vi "Connection Manager (general TDT).vi"(2 "Parent VI":refnum<vi>, 7 "AO Endpoints":string[](array[string])=["Right", "Left"], 9 "AI Endpoints":string[](array[string])=["Probe Mic Left", "Cal Mic"], 11 "error in (no error)":errorcluster) -> (4 "TDT-Device Config":T3, 6 "Properties":T2, 8 "Canceled?":bool, 15 "error out":errorcluster)   [LabVIEW 2020]
uses:
  Utility VIs/Buttons/KCheckmarkBoolean 2.ctl
  Utility VIs/Controls/KTable/KTable.xctl
  PXI DAQ VIs/TDT VIs/Typedefs/TDT-Device Config.ctl
  PXI DAQ VIs/TDT VIs/Typedefs/TDT-Output source.ctl
  PXI DAQ VIs/TDT VIs/Typedefs/TDT-Device ID.ctl
  PXI DAQ VIs/TDT VIs/Typedefs/TDT-Input source.ctl
  EPhys/LV Source/Typedefs/EPhys-Hardware Properties.ctl
panel:
  out "button":bool
  in  "Test Button":bool
  in  "Use kill switch":T1
  in  "Input Table":u16(xcontrol)
  in  "Path":path
  in  "Output Table":u16(xcontrol)
  in  "Biosemi":T1
  in  "Input":enum16{"Front panel", "RA4LI", "RA16LI"}(ring)
  out "Image":enum32{"None", "RX6", "RZ5", "RZ6"}(tab)
  in  "Input source":u16(ring) items=["Front panel", "RA4LI", "RA16LI"]
  in  "Run on":u16(ring) items=["RZ5"]
  in  "Cancel":bool
  in  "OK":bool
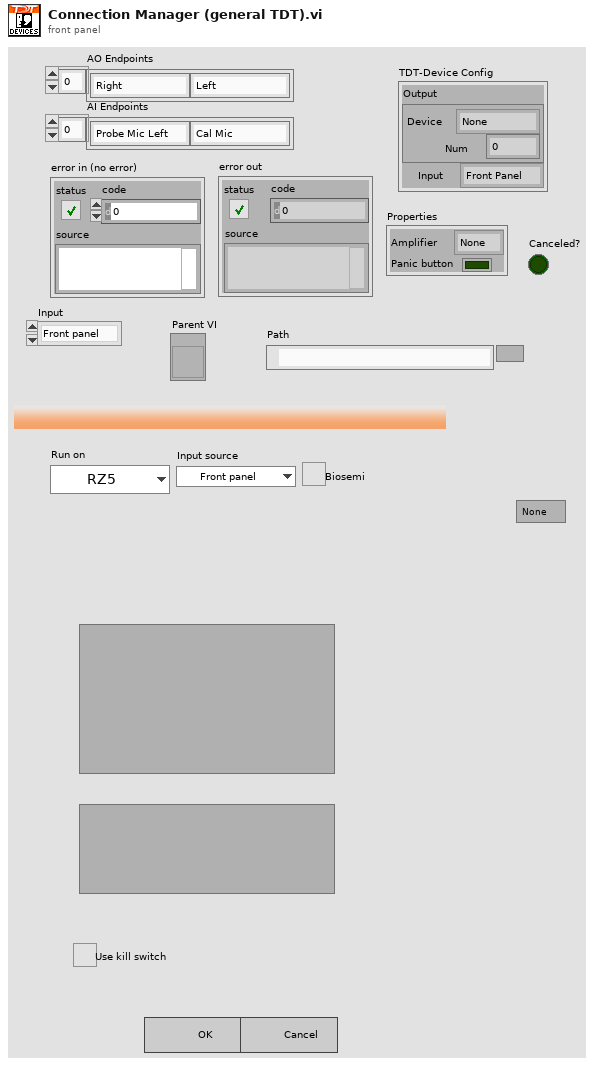
[diagram p1: front panel]
types:
  T1 = typedef "KCheckmarkBoolean 2.ctl" = bool
  T2 = typedef "EPhys-Hardware Properties.ctl" = cluster{"Amplifier":enum16{"None", "Biosemi", "Eclipse", "Eclipse (N.C.)", "Grass"}, "Panic button":bool}
  T3 = typedef "TDT-Device Config.ctl" = cluster{"Output":T4, "Input":T6}
  T4 = typedef "TDT-Output source.ctl" = cluster{"Device":T5, "Num":i32}
  T5 = typedef "TDT-Device ID.ctl" = enum16{"None", "PA5", "RP2", "RL2", "RA16", "RV8", "RX5", "RX6", "RX7", "RX8", "RZ2", "RZ5", "RZ6"}
  T6 = typedef "TDT-Input source.ctl" = enum16{"Front Panel", "RA4LI", "RA16LI"}
  T7 = enum16{"None", "Biosemi", "Eclipse", "Eclipse (N.C.)", "Grass"}
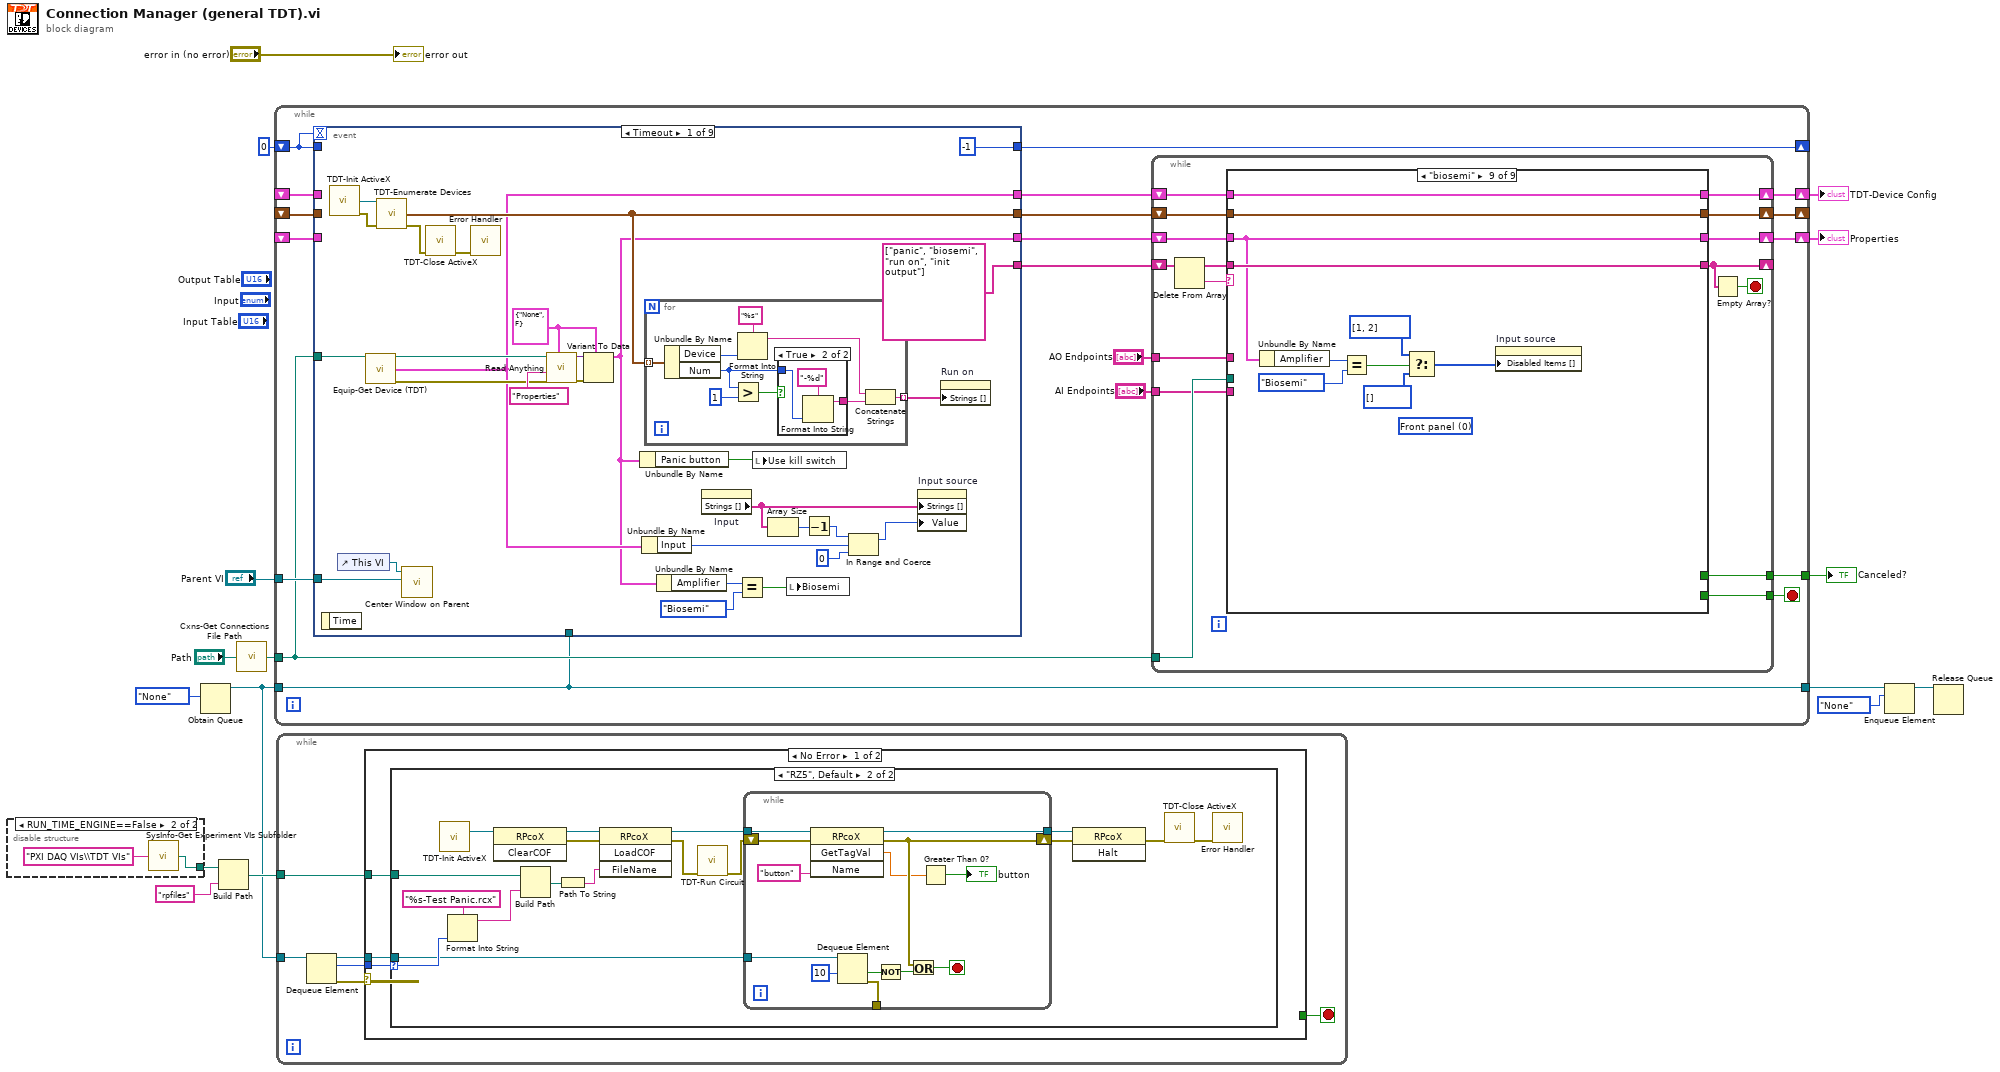
[diagram p0: block diagram]
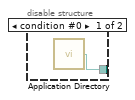
[diagram p2: hidden frame]
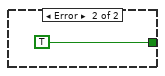
[diagram p4: hidden frame]
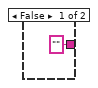
[diagram p5: hidden frame]
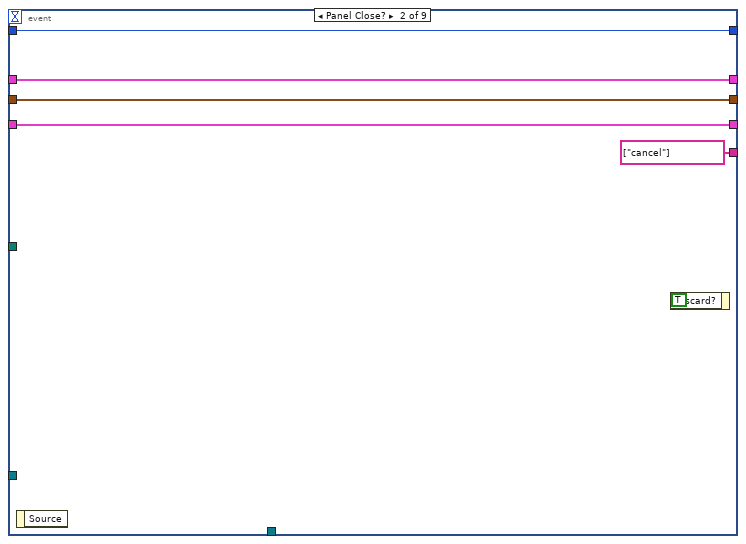
[diagram p6: hidden frame]
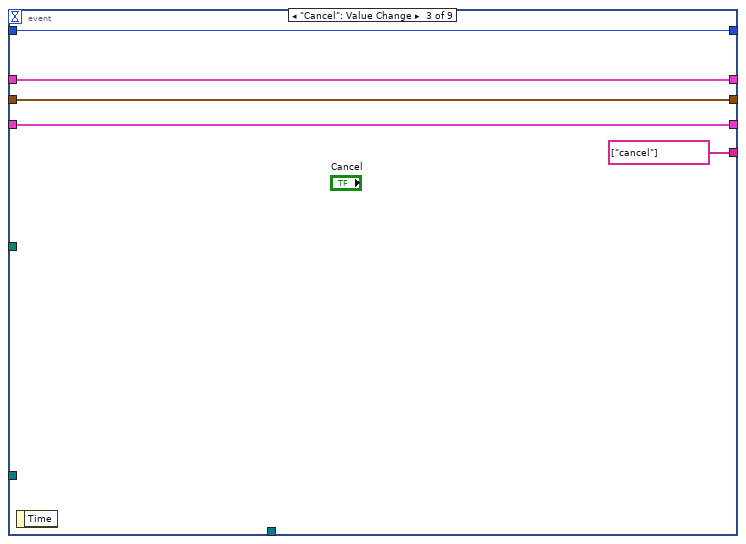
[diagram p7: hidden frame]
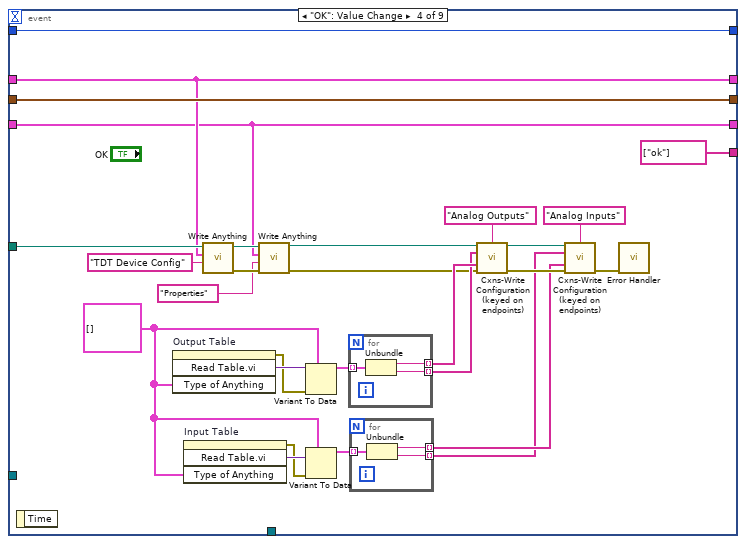
[diagram p8: hidden frame]
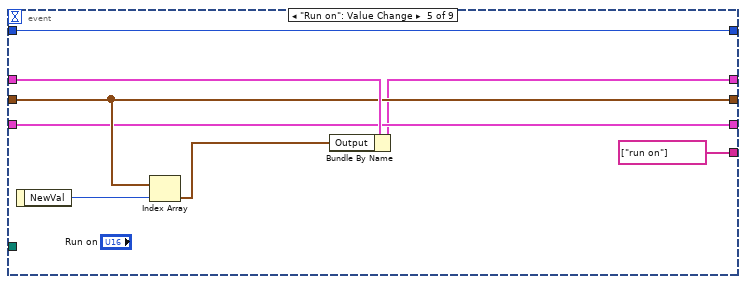
[diagram p9: hidden frame]
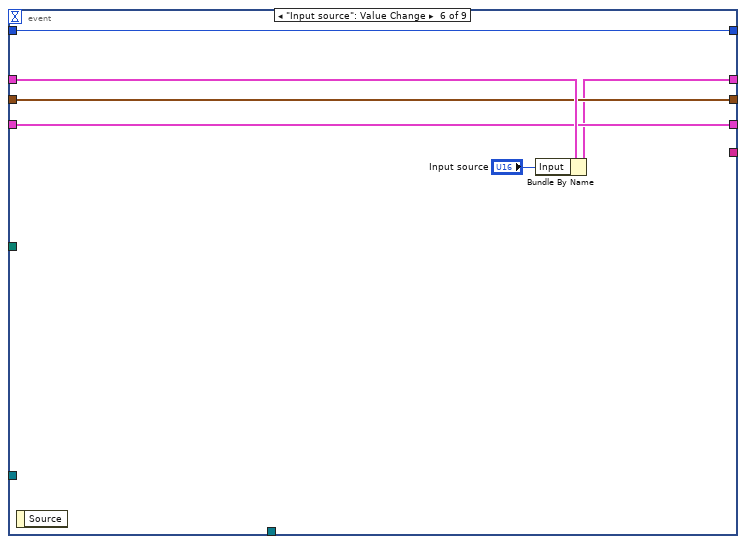
[diagram p10: hidden frame]
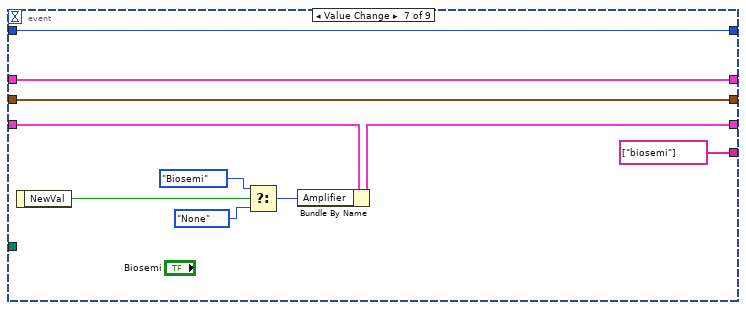
[diagram p11: hidden frame]
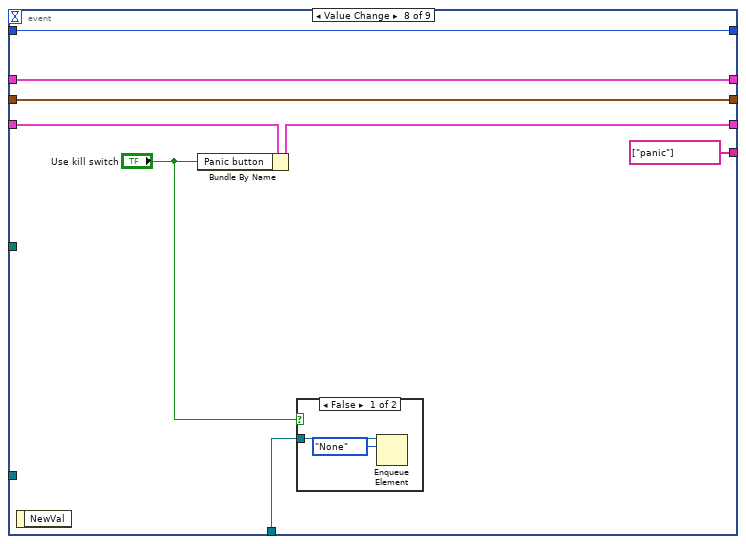
[diagram p12: hidden frame]
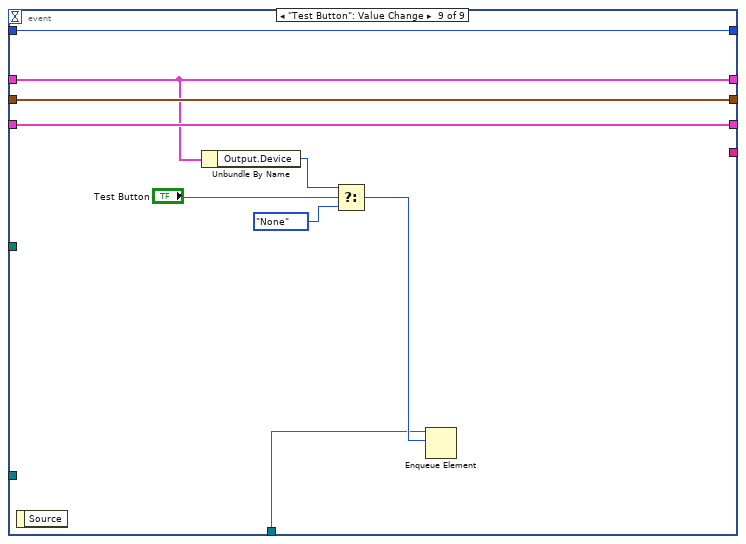
[diagram p14: hidden frame]
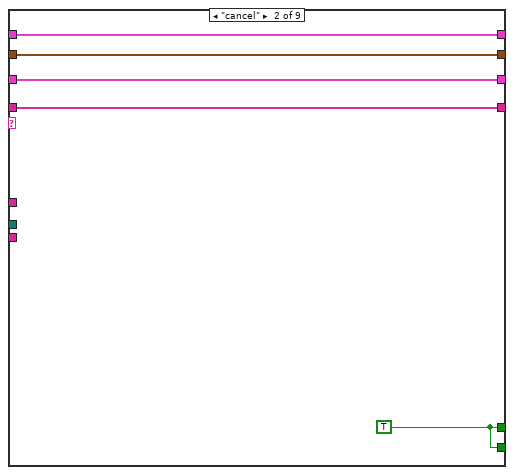
[diagram p16: hidden frame]
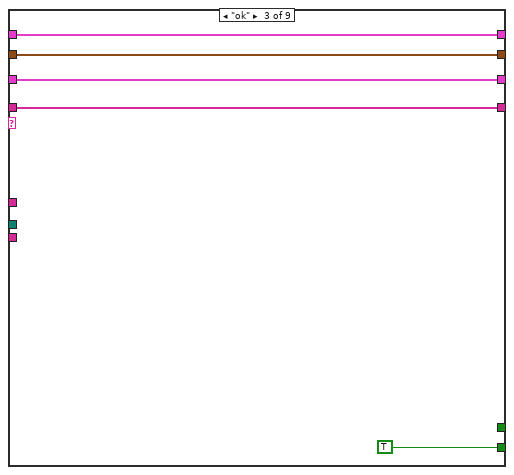
[diagram p17: hidden frame]
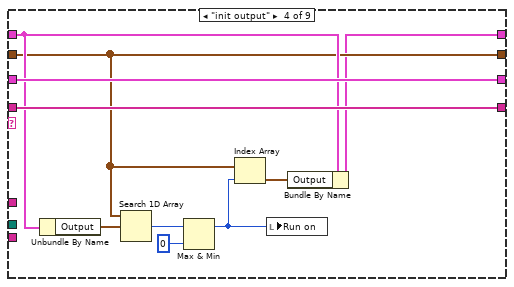
[diagram p18: hidden frame]
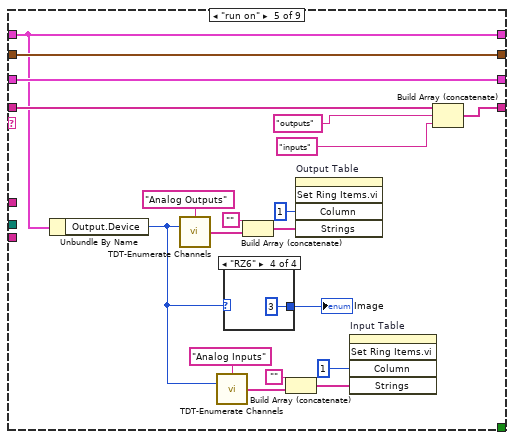
[diagram p19: hidden frame]
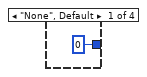
[diagram p20: hidden frame]
diagram:
  n1 = disable-structure shown="RUN_TIME_ENGINE==False" {
    disable-tunnel: [w17 w19] -> w7
    frame condition #0 {
      n2 = call <vilib>:"Application Directory.vi"() -> ("Application Directory"=w17:path)
    }
    frame condition #1 (active) {
      n3 = call "SysInfo-Get Experiment VIs Subfolder.vi"("subfolder"="PXI DAQ VIs\\TDT VIs") -> ("full path"=w19:path)  [unwired: 4 in]
    }
  }
  n4 = Obtain Queue(element data type=TDT-Device_ID."None" ("Output.Device")) -> (queue out=w4:refnum<queue>)  [unwired: 4 in, 2 out]
  n5 = Build Path(base path=w7, name or relative path="rpfiles") -> (appended path=w5:path)
  n6 = call "Cxns-Get Connections File Path.vi"("Connection File Path"="Path") -> ("Path Out"=w13:path)
  n7 = while {
    shift-right: [w38] -> _
    shift-left: 0 -> [w36]
    tunnel: [w25] -> w15
    shift-right: [w30] -> w10
    shift-left: _ -> [w37]
    shift-right: [w28] -> _
    shift-left: _ -> [w35]
    tunnel: "Parent VI" -> [w34]
    shift-right: [w26] -> w9
    shift-left: _ -> [w33]
    tunnel: w13 -> [w23]
    tunnel: w4 -> [w20]
    tunnel: [w20] -> w1
    stop <- w24 stop-if-true
    n8 = event shown="[0] Timeout" {
      selector: _ -> [_ _ _ _ _ _ _ _ _]
      dyn-events: _ -> [_ _ _ _ _ _ _ _ _]
      timeout: w36 -> [_ _ _ _ _ _ _ _ _]
      tunnel: [-1 w86 w91 w119 w133 w139 w149 w157 w168] -> w38
      tunnel: w37 -> [_ w85 w88 w115 w132 w138 w148 w156 w160]
      tunnel: [w43 w85 w88 w115 w128 w135 w148 w156 w160] -> w31
      tunnel: w36 -> [_ w86 w91 w119 w133 w139 w149 w157 w168]
      tunnel: [w65 w83 w90 w118 w131 w137 w147 w155 w167] -> w29
      tunnel: w35 -> [_ w83 w90 w118 w131 w137 w147 w155 w167]
      tunnel: w34 -> [w58 _ _ _ _ _ _ _ _]
      tunnel: w33 -> [_ w82 w87 w106 w129 w136 w146 w154 w166]
      tunnel: [w41 w82 w87 w106 w129 w136 w145 w153 w166] -> w27
      tunnel: w23 -> [w45 _ _ w116 _ _ _ _ _]
      tunnel: [string[] ["panic", "biosemi", "run on", "init output"] string[] ["cancel"] string[] ["cancel"] string[] ["ok"] string[] ["run on"] _ string[] ["biosemi"] string[] ["panic"] _] -> w32
      tunnel: w20 -> [_ _ _ _ _ _ _ w152 w162]
      event Timeout {
        w52 = T2 {"Amplifier"=enum."None", "Panic button"=FALSE} ("Properties In")
        n9 = event-data() -> ()  [unwired: 1 in, 1 out]
        n10 = call "TDT-Init ActiveX.vi"() -> ("ZBUSx"=w50:refnum<k7>, "error out"=w47:errorcluster)  [unwired: 12 in, 2 out]
        n11 = control-ref of="This VI"() -> (w57:refnum<vi>)
        n12 = call "Equip-Get Device (TDT).vi"("Path In"=w45) -> ("Path Out"=w44:path, "TDT-Device Config"=w43:T3, "error out"=w46:errorcluster)  [unwired: 12 in]
        n13 = call "TDT-Enumerate Devices.vi"("ZBUSx In"=w50, "error in (no error)"=w47) -> ("Devices"=w65:T4[], "error out"=w48:errorcluster)  [unwired: 11 in, 1 out]
        n14 = call "Center Window on Parent.vi"("Parent VI"=w58, "VI in"=w57) -> ()  [unwired: 8 in, 2 out]
        n15 = call "TDT-Close ActiveX.vi"("error in (no error)"=w48) -> ("error out"=w49:errorcluster)  [unwired: 14 in]
        n16 = call "Error Handler.vi"("error in (no error)"=w49) -> ()  [unwired: 13 in, 2 out]
        n17 = call "Read Anything.vi"("Type of Anything"=w52, "Error In"=w46, "Section Name (Name of \"Type of Anything\")"="Properties" ("Section Name (Name of \"Type of Anything\")"), "Path (dialog)"=w44) -> ("Error Out"=w54:errorcluster, "Anything"=w53:variant)  [unwired: 5 in, 1 out]
        n18 = Variant To Data(error in=w54, type=w52, Variant=w53) -> (data=w41:T2)  [unwired: 1 out]
        n19 = Unbundle By Name(w41) -> ("Panic button"=w40:bool)
        n20 = Unbundle By Name(w43) -> ("Input"=w60:T6)
        n21 = for {
          tunnel: w65 -> [w76] mode=indexing
          tunnel: [w70] -> w66 mode=indexing
          n22 = Unbundle By Name(w76) -> ("Device"=w68:T5, "Num"=w71:i32)
          n23 = Greater?(x=w71, y=1) -> (0:w72:bool)
          n24 = Format Into String(format string="%s", w68) -> (resulting string=w74:string)  [unwired: 2 in, 1 out]
          n25 = case shown="True" w72 {
            tunnel: w71 -> [_ w79]
            tunnel: ["" w78] -> w69
            frame False {
            }
            frame True {
              n26 = Format Into String(format string="-%d", w79) -> (resulting string=w78:string)  [unwired: 2 in, 1 out]
            }
          }
          n27 = Concatenate Strings(w74, w69) -> (w70:string)
        }
        n28 = Unbundle By Name(w41) -> ("Amplifier"=w56:T7)
        n29 = property on="Input" class="Enum (strict)"() -> ("Strings []"=w64:string[])  [unwired: 2 in, 2 out]
        n30 = Equal?(x=w56, y=T7."Biosemi") -> (x = y?=w55:bool)
        n31 = local write "Use kill switch"(w40) -> ()
        n32 = Array Size(array=w64) -> (size(s)=w63:i32)
        n33 = local write "Biosemi"(w55) -> ()
        n34 = Decrement(x=w63) -> (x-1=w62:i32)
        n35 = In Range and Coerce(upper limit=w62, x=w60, lower limit=0) -> (coerced(x)=w61:i32)  [unwired: 1 out]
        n36 = property on="Input source" class="Ring (strict)"("Strings []"=w64, "Value"=w61) -> ()  [unwired: 2 in, 2 out]
        n37 = property on="Run on" class="Ring (strict)"("Strings []"=w66) -> ()  [unwired: 2 in, 2 out]
      }
      event Panel Close? {
        n38 = event-data() -> ()  [unwired: 1 in, 1 out]
        n39 = event-data("Discard?"=TRUE) -> ()  [unwired: 1 in, 1 out]
      }
      event "Cancel": Value Change {
        n40 = event-data() -> ()  [unwired: 1 in, 1 out]
      }
      event "OK": Value Change {
        w97 = cluster{"IOChannel":string, "Endpoint":string}[] []
        n41 = event-data() -> ()  [unwired: 1 in, 1 out]
        n42 = invoke on="Output Table" class="KTable (strict)" method="Read Table.vi"("Type of Anything"=w97) -> (error out=w112:errorcluster, "Read Table.vi"=w113:variant)  [unwired: 3 in, 2 out]
        n43 = invoke on="Input Table" class="KTable (strict)" method="Read Table.vi"("Type of Anything"=w97) -> (error out=w98:errorcluster, "Read Table.vi"=w99:variant)  [unwired: 3 in, 2 out]
        n44 = call "Write Anything.vi"("Section Name (Name of \"Anything\")"="TDT Device Config" ("Section Name (Name of \"Anything\")"), "Anything"=w115, "Path (dialog)"=w116) -> ("Error Out"=w108:errorcluster, "Path out"=w107:path)  [unwired: 7 in]
        n45 = call "Write Anything.vi"("Error In"=w108, "Section Name (Name of \"Anything\")"="Properties" ("Section Name (Name of \"Anything\")"), "Anything"=w106, "Path (dialog)"=w107) -> ("Error Out"=w104:errorcluster, "Path out"=w103:path)  [unwired: 6 in]
        n46 = Variant To Data(error in=w112, type=w97, Variant=w113) -> (data=w111:cluster{"IOChannel":string, "Endpoint":string}[])  [unwired: 1 out]
        n47 = Variant To Data(error in=w98, type=w97, Variant=w99) -> (data=w96:cluster{"IOChannel":string, "Endpoint":string}[])  [unwired: 1 out]
        n48 = for {
          tunnel: w111 -> [w125] mode=indexing
          tunnel: [w124] -> w110 mode=indexing
          tunnel: [w123] -> w109 mode=indexing
          n49 = Unbundle(w125) -> ("IOChannel"=w124:string, "Endpoint"=w123:string)
        }
        n50 = for {
          tunnel: w96 -> [w122] mode=indexing
          tunnel: [w121] -> w95 mode=indexing
          tunnel: [w120] -> w94 mode=indexing
          n51 = Unbundle(w122) -> ("IOChannel"=w121:string, "Endpoint"=w120:string)
        }
        n52 = call "Cxns-Write Configuration (keyed on endpoints).vi"("Connection File Path"=w103, "Section"="Analog Outputs" ("format string"), "Outputs"=w109, "Endpoints"=w110, "error in (no error)"=w104) -> ("Path Out"=w102:path, "error out"=w101:errorcluster)  [unwired: 9 in]
        n53 = call "Cxns-Write Configuration (keyed on endpoints).vi"("Connection File Path"=w102, "Section"="Analog Inputs" ("format string"), "Outputs"=w94, "Endpoints"=w95, "error in (no error)"=w101) -> ("error out"=w100:errorcluster)  [unwired: 9 in, 1 out]
        n54 = call "Error Handler.vi"("error in (no error)"=w100) -> ()  [unwired: 13 in, 2 out]
      }
      event "Run on": Value Change {
        n55 = event-data() -> ("NewVal"=w130:u16)  [unwired: 1 in]
        n56 = Index Array(array=w131, index=w130) -> (element=w126:T4)
        n57 = Bundle By Name(cluster=w132, "Output"=w126) -> (w128:T3)
      }
      event "Input source": Value Change {
        n58 = event-data() -> ()  [unwired: 1 in, 1 out]
        n59 = Bundle By Name(cluster=w138, "Input"="Input source") -> (w135:T3)
      }
      event Value Change {
        n60 = event-data() -> ("NewVal"=w144:T1)  [unwired: 1 in]
        n61 = Select(t=T7."Biosemi" ("Amplifier"), s=w144, f=T7."None" ("Amplifier")) -> (s? t:f=w142:T7)
        n62 = Bundle By Name(cluster=w146, "Amplifier"=w142) -> (w145:T2)
      }
      event Value Change {
        n63 = event-data() -> ()  [unwired: 1 in, 1 out]
        n64 = Bundle By Name(cluster=w154, "Panic button"="Use kill switch") -> (w153:T2)
        n65 = case shown="False" "Use kill switch" {
          tunnel: w152 -> [w159 _]
          frame False {
            n66 = Enqueue Element(queue=w159, element=TDT-Device_ID."None") -> ()  [unwired: 2 in, 3 out]
          }
          frame True {
          }
        }
      }
      event "Test Button": Value Change {
        n67 = event-data() -> ()  [unwired: 1 in, 1 out]
        n68 = Unbundle By Name(w160) -> ("Output.Device"=w163:T5)
        n69 = Select(t=w163, s="Test Button", f=TDT-Device_ID."None") -> (s? t:f=w165:T5)
        n70 = Enqueue Element(queue=w162, element=w165) -> ()  [unwired: 2 in, 3 out]
      }
    }
    n71 = while {
      shift-right: [w181] -> _
      shift-left: w32 -> [w184]
      shift-right: [w178] -> w30
      shift-left: w31 -> [w179]
      shift-right: [w176] -> w28
      shift-left: w29 -> [w177]
      shift-right: [w174] -> w26
      shift-left: w27 -> [w175]
      tunnel: [w173] -> w25
      tunnel: [w172] -> w24
      tunnel: w23 -> [w171]
      tunnel: "AO Endpoints" -> [w170]
      tunnel: "AI Endpoints" -> [w169]
      stop <- w180 stop-if-true
      n72 = Delete From Array(array=w184) -> (deleted portion=w182:string, array with subset deleted=w183:string[])  [unwired: 2 in]
      n73 = case shown="\"biosemi\"" w182 {
        tunnel: w183 -> [w188 w193 w198 w208 w227 w237 w247 w260 w273]
        tunnel: [w188 w193 w198 w208 w219 w237 w247 w260 w273] -> w181
        tunnel: w179 -> [w187 w192 w197 w203 w222 w236 w242 w255 w272]
        tunnel: [w187 w192 w197 w200 w222 w236 w242 w255 w272] -> w178
        tunnel: w177 -> [w186 w191 w196 w202 w226 w235 w246 w259 w271]
        tunnel: [w186 w191 w196 w202 w226 w235 w246 w259 w271] -> w176
        tunnel: w175 -> [w185 w190 w195 w207 w225 w232 w245 w258 w267]
        tunnel: [w185 w190 w195 w207 w225 w232 w245 w258 w267] -> w174
        tunnel: [_ w189 _ _ _ _ _ _ _] -> w173
        tunnel: [_ w189 TRUE _ _ _ _ _ _] -> w172
        tunnel: w171 -> [_ _ _ _ _ _ w243 w256 _]
        tunnel: w170 -> [_ _ _ _ _ _ w241 _ _]
        tunnel: w169 -> [_ _ _ _ _ _ _ w252 _]
        frame "", Default {
        }
        frame "cancel" {
          w189 = TRUE
        }
        frame "ok" {
        }
        frame "init output" {
          n74 = Unbundle By Name(w203) -> ("Output"=w204:T4)
          n75 = Search 1D Array(1D array=w202, element=w204) -> (index of element=w205:i32)  [unwired: 1 in]
          n76 = Max & Min(x=w205, y=0) -> (max(x,y)=w201:i32)  [unwired: 1 out]
          n77 = Index Array(array=w202, index=w201) -> (element=w199:T4)
          n78 = local write "Run on"(w201) -> ()
          n79 = Bundle By Name(cluster=w203, "Output"=w199) -> (w200:T3)
        }
        frame "run on" {
          n80 = Unbundle By Name(w222) -> ("Output.Device"=w211:T5)
          n81 = call "TDT-Enumerate Channels.vi"("Type"="Analog Outputs", "IO Device"=w211) -> ("IO Channels"=w220:string[])  [unwired: 13 in]
          n82 = call "TDT-Enumerate Channels.vi"("Type"="Analog Inputs", "IO Device"=w211) -> ("IO Channels"=w213:string[])  [unwired: 13 in]
          n83 = case shown="\"RZ6\"" w211 {
            tunnel: [0 1 2 3] -> w223
            frame "None", Default {
            }
            frame "RX6" {
            }
            frame "RZ5" {
            }
            frame "RZ6" {
            }
          }
          "Image" <- w223
          n84 = Build Array (concatenate)("", w220) -> (w217:string[])
          n85 = Build Array (concatenate)("", w213) -> (w209:string[])
          n86 = invoke on="Output Table" class="KTable (strict)" method="Set Ring Items.vi"("Column"=1, "Strings"=w217) -> ()  [unwired: 3 in, 5 out]
          n87 = invoke on="Input Table" class="KTable (strict)" method="Set Ring Items.vi"("Column"=1, "Strings"=w209) -> ()  [unwired: 3 in, 5 out]
          n88 = Build Array (concatenate)(w227, "outputs", "inputs") -> (w219:string[])
        }
        frame "panic" {
          n89 = Unbundle By Name(w232) -> ("Panic button"=w233:bool)
          n90 = property on="Test Button" class="Bool (strict)"("Visible"=w233) -> ()  [unwired: 2 in, 2 out]
          n91 = property on="button" class="Bool (strict)"("Visible"=w233, "Value"=FALSE ("button")) -> ()  [unwired: 2 in, 2 out]
        }
        frame "outputs" {
          n92 = call "Cxns-Read Configuration.vi"("Connection File Path"=w243, "Section"="Analog Outputs" ("format string"), "Outputs"=w241) -> ("Endpoints"=w240:string[])  [unwired: 11 in, 1 out]
          n93 = for {
            tunnel: w241 -> [w250] mode=indexing
            tunnel: w240 -> [w249] mode=indexing
            tunnel: [w248] -> w239 mode=indexing
            n94 = Bundle("String"=w250, "String"=w249) -> (w248:cluster{"String":string, "String":string})  [unwired: 1 in]
          }
          n95 = control-ref of="Output Table"() -> (w244:refnum<vi>)
          n96 = property class="KTable (strict)"(reference=w244, "Table"=w239) -> ()  [unwired: 1 in, 2 out]
        }
        frame "inputs" {
          n97 = call "Cxns-Read Configuration.vi"("Connection File Path"=w256, "Section"="Analog Inputs" ("format string"), "Outputs"=w252) -> ("Endpoints"=w254:string[])  [unwired: 11 in, 1 out]
          n98 = for {
            tunnel: w252 -> [w263] mode=indexing
            tunnel: w254 -> [w262] mode=indexing
            tunnel: [w261] -> w253 mode=indexing
            n99 = Bundle("String"=w263, "String"=w262) -> (w261:cluster{"String":string, "String":string})  [unwired: 1 in]
          }
          n100 = control-ref of="Input Table"() -> (w257:refnum<vi>)
          n101 = property class="KTable (strict)"(reference=w257, "Table"=w253) -> ()  [unwired: 1 in, 2 out]
        }
        frame "biosemi" {
          (unwired) u16 0 items=["Front panel", "RA4LI", "RA16LI"] ("Input source")
          n102 = Unbundle By Name(w267) -> ("Amplifier"=w266:T7)
          n103 = Equal?(x=w266, y=T7."Biosemi") -> (x = y?=w265:bool)
          n104 = Select(t=i32[] [1, 2], s=w265, f=i32[] [] ("Disabled Items []")) -> (s? t:f=w269:i32[])
          n105 = property on="Input source" class="Ring (strict)"("Disabled Items []"=w269) -> ()  [unwired: 2 in, 2 out]
        }
      }
      n106 = Empty Array?(array=w181) -> (empty?=w180:bool)
    }
  }
  "Canceled?" <- w15
  "TDT-Device Config" <- w10
  "Properties" <- w9
  n107 = while {
    tunnel: w4 -> [w279]
    tunnel: w5 -> [w276]
    stop <- w277 stop-if-true
    n108 = Dequeue Element(queue=w279) -> (queue out=w274:refnum<queue>, element=w275:T5, error out=w278:errorcluster)  [unwired: 2 in, 1 out]
    n109 = case shown="No Error" w278 {
      tunnel: [_ TRUE] -> w277
      tunnel: w276 -> [w281 _]
      tunnel: w275 -> [w282 _]
      tunnel: w274 -> [w280 _]
      frame No Error {
        n110 = case shown="\"RZ5\", Default" w282 {
          selector: w282 -> [_ w296]
          tunnel: w281 -> [_ w294]
          tunnel: w280 -> [_ w290]
          frame "None" {
          }
          frame "RZ5", Default {
            n111 = call "TDT-Init ActiveX.vi"() -> ("RPcox"=w285:refnum<k7>)  [unwired: 12 in, 3 out]
            n112 = Format Into String(format string="%s-Test Panic.rcx", w296) -> (resulting string=w295:string)  [unwired: 2 in, 1 out]
            n113 = invoke class="RPcoX" method="ClearCOF"(reference=w285) -> (reference out=w299:refnum<k7>, error out=w298:errorcluster)  [unwired: 2 in, 1 out]
            n114 = Build Path(base path=w294, name or relative path=w295) -> (appended path=w293:path)
            n115 = Path To String(path=w293) -> (string=w292:string)
            n116 = invoke class="RPcoX" method="LoadCOF"(reference=w299, error in=w298, "FileName"=w292) -> (reference out=w288:refnum<k7>, error out=w291:errorcluster)  [unwired: 1 in, 2 out]
            n117 = call "TDT-Run Circuit.vi"("error in (no error)"=w291) -> ("error out"=w289:errorcluster)  [unwired: 14 in]
            n118 = while {
              tunnel: w290 -> [w312]
              shift-right: [w304] -> w286
              shift-left: w289 -> [w305]
              tunnel: w288 -> [w306]
              tunnel: [w302] -> w287
              tunnel: [w301] -> _
              stop <- w308 stop-if-true
              n119 = invoke class="RPcoX" method="GetTagVal"(reference=w306, error in=w305, "Name"="button" ("format string")) -> (reference out=w302:refnum<k7>, error out=w304:errorcluster, "GetTagVal"=w303:sgl)  [unwired: 1 in, 1 out]
              n120 = Dequeue Element(queue=w312, timeout in ms (-1)=10) -> (timed out?=w310:bool, error out=w301:errorcluster)  [unwired: 1 in, 2 out]
              n121 = Not(x=w310) -> (.not. x?=w309:bool)
              n122 = Or(x=w304, y=w309) -> (x .or. y?=w308:bool)
              n123 = Greater Than 0?(x=w303) -> (x > 0?=→"button":bool)
            }
            n124 = invoke class="RPcoX" method="Halt"(reference=w287, error in=w286) -> (error out=w284:errorcluster)  [unwired: 1 in, 2 out]
            n125 = call "TDT-Close ActiveX.vi"("error in (no error)"=w284) -> ("error out"=w283:errorcluster)  [unwired: 14 in]
            n126 = call "Error Handler.vi"("error in (no error)"=w283) -> ()  [unwired: 13 in, 2 out]
          }
        }
      }
      frame Error {
      }
    }
  }
  n127 = Enqueue Element(queue=w1, element=TDT-Device_ID."None") -> (queue out=w2:refnum<queue>)  [unwired: 2 in, 2 out]
  n128 = Release Queue(queue=w2) -> ()  [unwired: 2 in, 3 out]
  "error out" <- "error in (no error)"
